vi "Actor Core.vi"(8 "error in":errorcluster, 11 "Hardware in":refnum<class "Hardware_panel.lvclass">) -> (0 "error out":errorcluster, 3 "Actor out":refnum<class "Actor.lvclass">)   [LabVIEW 2015, in "Hardware_panel.lvclass"]
doc: "(<B>Filename</B>: Actor Framework.lvlib:Actor.lvclass:Actor Core.vi)\n\nReceives messages to the actor, reacts to them, and initiates any error handling that may shut the actor down.\n\nDescendant classes may override this VI to append parallel tasks for the actor to complete while it handles messages. Overrides use the Call Parent Method node."
uses:
  Hardware_panel.lvclass
  <vilib>/ActorFramework/Actor/Actor.lvclass
  UI/panel_class/panel.lvclass/panel.ctl
  UI/panel_class/panel.lvclass
panel:
  # "Default Hardware"
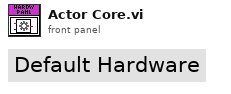
[diagram p1: front panel]
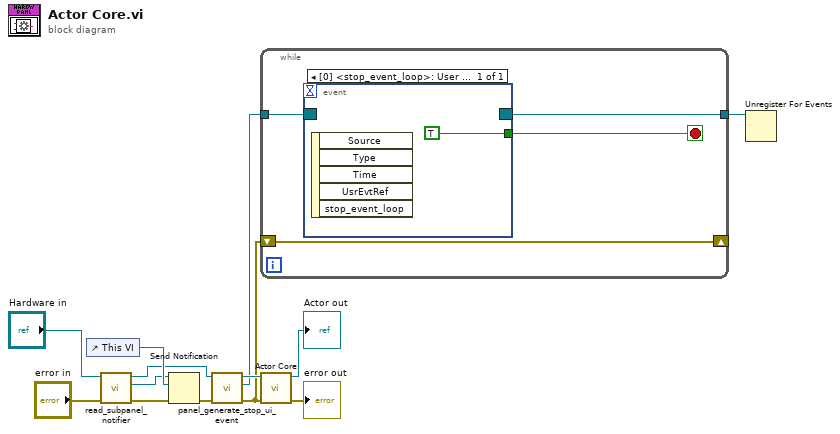
[diagram p0: block diagram]
diagram:
  n1 = control-ref of="This VI"() -> (w11:refnum<vi>)
  n2 = call "read_subpanel_notifier.vi"("error in (no error)"="error in", "panel in"="Hardware in") -> ("error out"=w7:errorcluster, "subpanel_notifier"=w9:refnum<notifier>, "panel out"=w8:refnum<class "Hardware_panel.lvclass">)  [unwired: 7 in]
  n3 = Send Notification(notification=w11, notifier=w9, error in (no error)=w7) -> (error out=w6:errorcluster)  [unwired: 1 out]
  n4 = call "panel_generate_stop_ui_event.vi"("error in (no error)"=w6, "panel in"=w8) -> ("error out"=w1:errorcluster, "stop_ui_ref"=w3:refnum<event-registration>, "panel out"=w5:refnum<class "Hardware_panel.lvclass">)  [unwired: 7 in]
  n5 = while {
    tunnel: w3 -> [w17]
    tunnel: [w15] -> w2
    shift-right: [w14] -> _
    shift-left: w1 -> [w14]
    stop <- w16 stop-if-true
    n6 = event shown="[0] <stop_event_loop>: User Event" {
      selector: w17 -> [_]
      dyn-events: [_] -> w15
      timeout: _ -> [_]
      tunnel: [TRUE] -> w16
      event User Event {
        n7 = event-data() -> ()  [unwired: 1 in, 5 out]
      }
    }
  }
  n8 = call-parent "Actor Core.vi"("error in"=w1, "Actor in"=w5) -> ("error out"=→"error out":errorcluster, "Actor out"=→"Actor out":refnum<class "Actor.lvclass">)  [unwired: 8 in]
  n9 = Unregister For Events(event registration refnum=w2) -> ()  [unwired: 1 in, 1 out]
